vi "Get Motor Angles.vi"(8 "error in (no error)":errorcluster, 11 "MF3 in":refnum<class "MF3.lvclass">) -> (0 "error out":errorcluster, 2 "motor angles":dbl[](array[numeric]) format="%.2f", 3 "MF3 out":refnum<class "MF3.lvclass">)   [LabVIEW 2013, in "MF3.lvclass"]
uses:
  MF3.lvclass
  MF3.lvclass/MF3.ctl
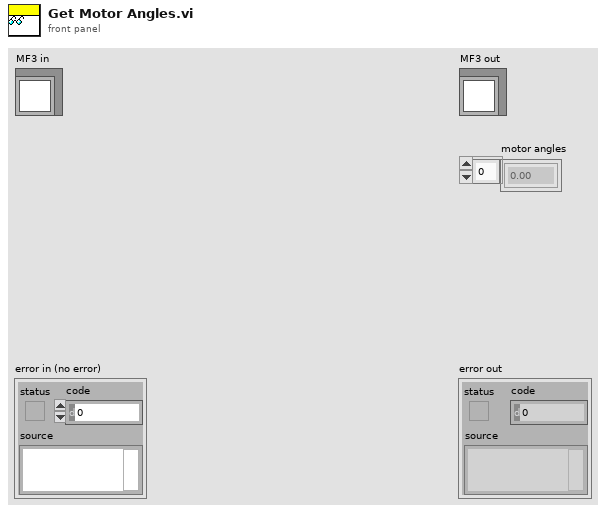
[diagram p1: front panel]
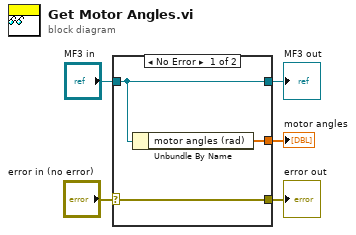
[diagram p0: block diagram]
diagram:
  n1 = case shown="No Error" "error in (no error)" {
    selector: "error in (no error)" -> [w8 w9]
    tunnel: [w8 w9] -> w4
    tunnel: [w7 w10] -> w2
    tunnel: "MF3 in" -> [w7 w10]
    tunnel: [w6 _] -> w1
    frame No Error {
      n2 = Unbundle By Name(w7) -> ("motor angles (rad)"=w6:dbl[])
    }
    frame Error {
    }
  }
  "error out" <- w4
  "MF3 out" <- w2
  "motor angles" <- w1
